vi "caminit.vi"(7 "error in (no error)":errorcluster, 10 "Camera Index":u32) -> (0 "error out":errorcluster, 1 "Cam Info":T1, 2 "Ranges":T3, 3 "Handle out":u32)   [LabVIEW 2015]
uses:
  <vilib>/Utility/miscctls.llb/LVMinMaxIncTypeDef.ctl
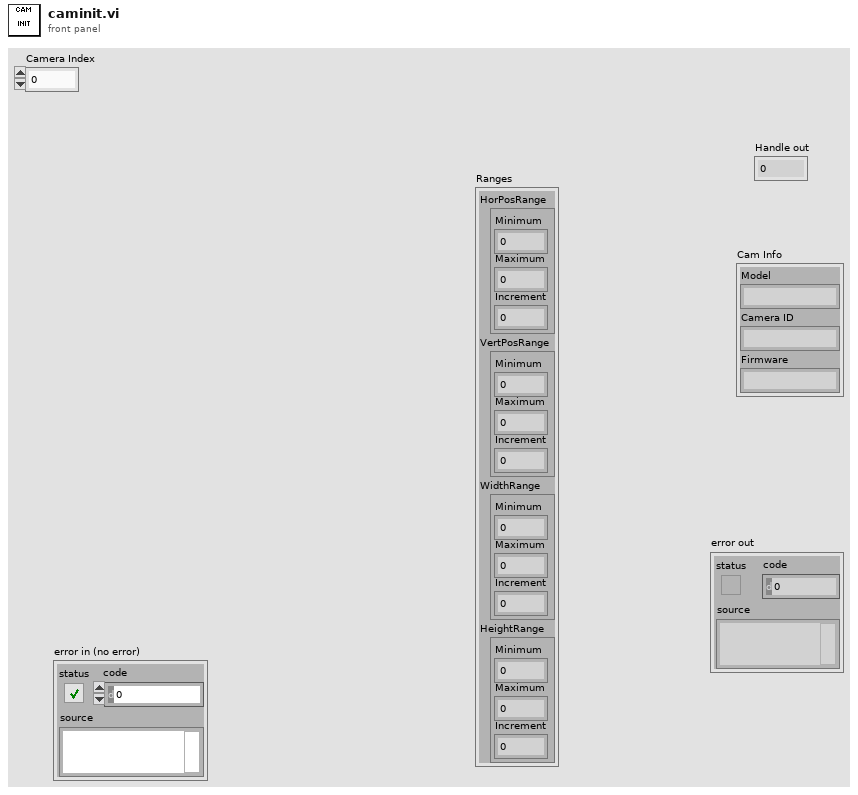
[diagram p1: front panel]
types:
  T1 = cluster{"Model":string, "Camera ID":string, "Firmware":string}
  T2 = typedef "LVMinMaxIncTypeDef.ctl" = cluster{"Minimum":dbl, "Maximum":dbl, "Increment":dbl}
  T3 = cluster{"HorPosRange":T2, "VertPosRange":T2, "WidthRange":T2, "HeightRange":T2}
  T4 = cluster{"H Offset":cluster{"Value":i32, "Limits":T2}, "V Offset":cluster{"Value":i32, "Limits":T2}, "H Size":cluster{"Value":i32, "Limits":T2}, "V Size":cluster{"Value":i32, "Limits":T2}}
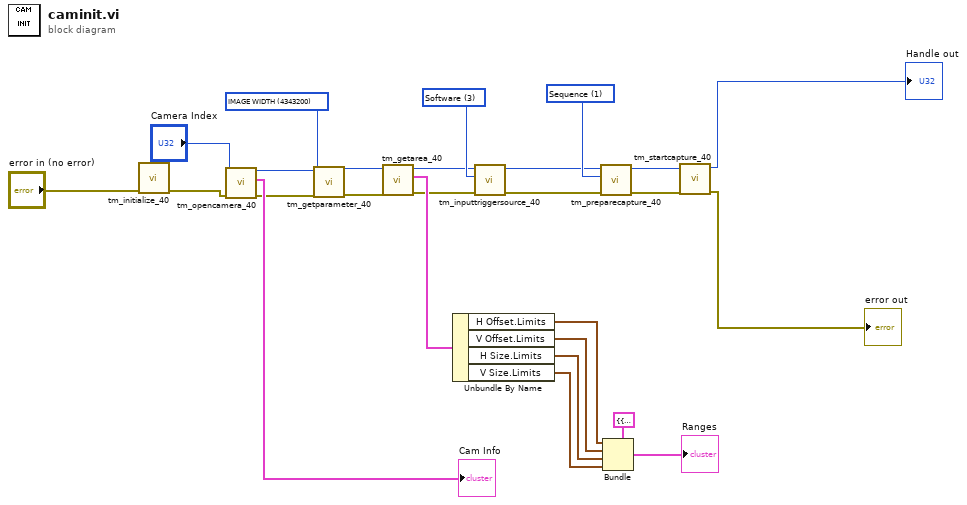
[diagram p0: block diagram]
diagram:
  w9 = 3 items=["Internal"=1, "External"=2, "Software"=3, "Master Pulse"=4] ("Source")
  w10 = 1 items=["Snap", "Sequence"] ("Capture mode")
  w22 = u32 4343200 items=["SENSOR MODE"=4212128, "READOUT SPEED"=4211872, "READOUT DIRECTION"=4211904, "TRIGGER GLOBAL EXPOSURE"=2049680, "TRIGGER DELAY"=1066480, "INTERNAL TRIGGER HANDLING"=1066496, "SENSOR TEMPERATURE"=2115232, "SENSOR COOLER STATUS"=2115280, "EXPOSURE TIME"=2049184, "DEFECT CORRECT MODE"=4670368, "HOT PIXEL CORRECT LEVEL"=4670400, "BINNING"=4215968, "TIMING READOUT TIME"=4223904, "INTERNAL FRAME RATE"=4225952, "INTERNAL FRAME INTERVAL"=4225968, "INTERNAL LINE SPEED"=4226000, "INTERNAL LINE INTERVAL"=4226016, "IMAGE WIDTH"=4343200, "IMAGE HEIGHT"=4343216, "IMAGE ROWBYTES"=4343232, "IMAGE FRAMEBYTES"=4343248, "IMAGE PIXEL TYPE"=4343296, "NUMBER OF OUTPUT TRIGGER CONNECTOR"=1852320, "OUTPUT TRIGGER SOURCE[0]"=1852576, "OUTPUT TRIGGER SOURCE[1]"=1852832, "OUTPUT TRIGGER SOURCE[2]"=1853088, "OUTPUT TRIGGER POLARITY[0]"=1852592, "OUTPUT TRIGGER POLARITY[1]"=1852848, "OUTPUT TRIGGER POLARITY[2]"=1853104, "OUTPUT TRIGGER ACTIVE[0]"=1852608, "OUTPUT TRIGGER ACTIVE[1]"=1852864, "OUTPUT TRIGGER ACTIVE[2]"=1853120, "OUTPUT TRIGGER DELAY[0]"=1852624, "OUTPUT TRIGGER DELAY[1]"=1852880, "OUTPUT TRIGGER DELAY[2]"=1853136, "OUTPUT TRIGGER PERIOD[0]"=1852640, "OUTPUT TRIGGER PERIOD[1]"=1852896, "OUTPUT TRIGGER PERIOD[2]"=1853152, "OUTPUT TRIGGER KIND[0]"=1852656, "OUTPUT TRIGGER KIND[1]"=1852912, "OUTPUT TRIGGER KIND[2]"=1853168, "OUTPUT TRIGGER BASE SENSOR[0]"=1852672, "OUTPUT TRIGGER BASE SENSOR[1]"=1852928, "OUTPUT TRIGGER BASE SENSOR[2]"=1853184, "OUTPUT TRIGGER PRE HSYNC COUNT"=1852704] ("Parameter")
  n1 = call <userlib>:"tm_initialize_40.vi"("error in (no error)"="error in (no error)") -> ("error out"=w25:errorcluster)  [unwired: 7 in, 3 out]
  n2 = call <userlib>:"tm_opencamera_40.vi"("error in (no error)"=w25, "Camera Index"="Camera Index") -> ("error out"=w12:errorcluster, "Camera Details"=→"Cam Info":T1, "Handle out"=w23:u32)  [unwired: 7 in]
  n3 = call <userlib>:"tm_getparameter_40.vi"("error in (no error)"=w12, "Parameter"=w22, "Handle in"=w23) -> ("error out"=w11:errorcluster, "Handle out"=w20:u32)  [unwired: 6 in, 1 out]
  n4 = call <userlib>:"tm_getarea_40.vi"("error in (no error)"=w11, "Handle in"=w20) -> ("error out"=w7:errorcluster, "Sub Region"=w19:T4, "Handle out"=w8:u32)  [unwired: 7 in]
  n5 = Unbundle By Name(w19) -> ("H Offset.Limits"=w17:T2, "V Offset.Limits"=w16:T2, "H Size.Limits"=w15:T2, "V Size.Limits"=w14:T2)
  n6 = call <userlib>:"tm_inputtriggersource_40.vi"("error in (no error)"=w7, "Source"=w9, "Handle in"=w8) -> ("error out"=w6:errorcluster, "Handle out"=w5:u32)  [unwired: 7 in]
  n7 = call <userlib>:"tm_preparecapture_40.vi"("error in (no error)"=w6, "Capture mode"=w10, "Handle in"=w5) -> ("error out"=w4:errorcluster, "Handle out"=w2:u32)  [unwired: 5 in, 2 out]
  n8 = Bundle(cluster=T3 {"HorPosRange"={"Minimum"=0.0, "Maximum"=0.0, "Increment"=0.0}, "VertPosRange"={"Minimum"=0.0, "Maximum"=0.0, "Increment"=0.0}, "WidthRange"={"Minimum"=0.0, "Maximum"=0.0, "Increment"=0.0}, "HeightRange"={"Minimum"=0.0, "Maximum"=0.0, "Increment"=0.0}} ("Ranges 2"), "HorPosRange"=w17, "VertPosRange"=w16, "WidthRange"=w15, "HeightRange"=w14) -> (→"Ranges":T3)
  n9 = call <userlib>:"tm_startcapture_40.vi"("error in (no error)"=w4, "Handle in"=w2) -> ("error out"=→"error out":errorcluster, "Handle out"=→"Handle out":u32)  [unwired: 8 in]
